vi "Add Trace Log.vi"(5 "Info":string, 7 "LabVIEW Object":refnum<class>, 10 "error in (no error)":errorcluster, 11 "Processing in":refnum<class "Processing.lvclass">) -> (2 "error out":errorcluster, 3 "Processing out":refnum<class "Processing.lvclass">)   [LabVIEW 2020, in "HTTP Server.lvlib" / "Processing.lvclass"]
uses:
  Processing.lvclass
  Processing.lvclass/Processing.ctl
  RequestTraceLog/RequestTraceLog.lvclass
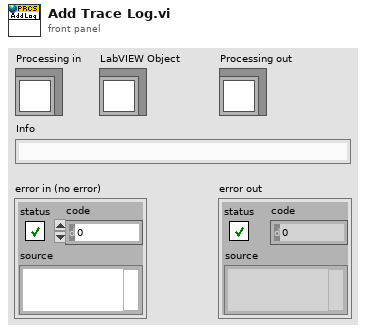
[diagram p1: front panel]
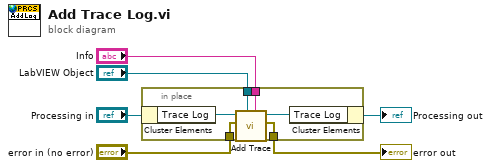
[diagram p0: block diagram]
diagram:
  n1 = in-place {
    in-place-border: "LabVIEW Object" -> [w12]
    in-place-border: "Info" -> [w11]
    in-place-border: "error in (no error)" -> [w10]
    in-place-border: [w9] -> w3
    n2 = in-place-cluster #1("Processing in") -> ("Trace Log"=w8:refnum<class "RequestTraceLog.lvclass">)
    n3 = call "Add Trace.vi"("Info"=w11, "LabVIEW Object"=w12, "error in (no error)"=w10, "RequestTraceLog in"=w8) -> ("error out"=w9:errorcluster, "RequestTraceLog out"=w7:refnum<class "RequestTraceLog.lvclass">)  [unwired: 6 in]
    n4 = in-place-cluster #1("Trace Log"=w7) -> (→"Processing out":refnum<class "Processing.lvclass">)
  }
  "error out" <- w3
